vi "Write Report.vi"(8 "error in (no error)":errorcluster, 10 "Resource In":variant, 11 "Analyze Parameter Temporal Calibration in":refnum<class "Analyze Parameter Temporal Calibration.lvclass">) -> (0 "error out":errorcluster, 2 "Resource Out":variant, 3 "Analyze Parameter Temporal Calibration out":refnum<class "Analyze Parameter Temporal Calibration.lvclass">)   [LabVIEW 2020, in "Analyze Parameter Temporal Calibration.lvclass"]
uses:
  Analyze Parameter Temporal Calibration.lvclass
  C:/POLARIS Programme/POLARIS-AS-3-Cams/Submodules/HIJ Vision/Analyze/Analyze Parameter/Analyze Parameter Base/Analyze Parameter Base.lvclass
  <vilib>/Utility/config.llb/Config Data RefNum.ctl
  Analyze Parameter Temporal Calibration.lvclass/Analyze Parameter Temporal Calibration.ctl
  <vilib>/Utility/config.llb/Write Key (Double).vi
  <vilib>/Utility/config.llb/NI_LVConfig.lvlib
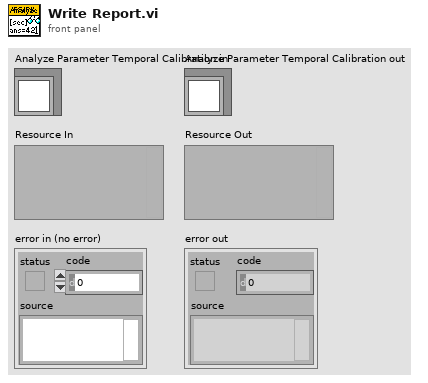
[diagram p1: front panel]
types:
  T1 = typedef "NI_LVConfig.lvlib/Config Data RefNum.ctl" = refnum<k1>
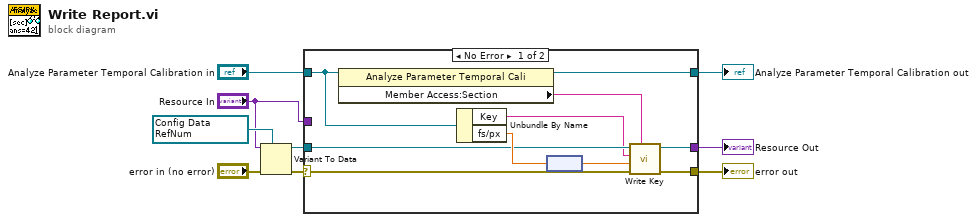
[diagram p0: block diagram]
diagram:
  w9 = T1 refnum items=["config data"] ("refnum")
  n1 = Variant To Data(error in="error in (no error)", type=w9, Variant="Resource In") -> (data=w3:T1, error out=w1:errorcluster)
  n2 = case shown="No Error" w1 {
    selector: w1 -> [w16 w21]
    tunnel: w3 -> [w15 _]
    tunnel: "Analyze Parameter Temporal Calibration in" -> [w18 w20]
    tunnel: [w19 w20] -> w6
    tunnel: [w14 w22] -> w5
    tunnel: [w13 w21] -> w4
    tunnel: "Resource In" -> [_ w22]
    frame No Error {
      n3 = property class="Analyze Parameter Temporal Cali"(reference=w18) -> (reference out=w19:refnum<class "Analyze Parameter Temporal Calibration.lvclass">, "Member Access:Section"=w10:string)  [unwired: 1 in, 1 out]
      n4 = Unbundle By Name(w18) -> ("Key"=w12:string, "fs/px"=w17:dbl[unit])
      n5 = node(w17) -> (w11:dbl)
      n6 = call-poly <vilib>:"Write Key.vi"("section"=w10, "error in (no error)"=w16, "value"=w11, "key"=w12, "refnum"=w15) -> ("error out"=w13:errorcluster, "refnum out"=w14:T1)  [unwired: 4 in, 1 out]
    }
    frame Error {
    }
  }
  "error out" <- w4
  "Analyze Parameter Temporal Calibration out" <- w6
  "Resource Out" <- w5
